vi "Pre Launch Init.vi"(11 "Measurement Señal Actualizable in":refnum<class "Measurement Señal Actualizable.lvclass">) -> (0 "error out":errorcluster, 3 "Measurement Señal Actualizable out":refnum<class "Measurement Señal Actualizable.lvclass">)   [LabVIEW 2020, in "Measurement Señal Actualizable.lvlib" / "Measurement Señal Actualizable.lvclass"]
doc: "(<B>Filename</B>: Actor Framework.lvlib:Actor.lvclass:Pre Launch Init.vi)\n\nDefines behavior that occurs after the Launch Nested Actor method is invoked but before the actor's Actor Core method begins running.\n\nBy default, this method does nothing. A descendant class may override it to define behavior."
uses:
  <vilib>/ActorFramework/Actor/Actor.lvclass
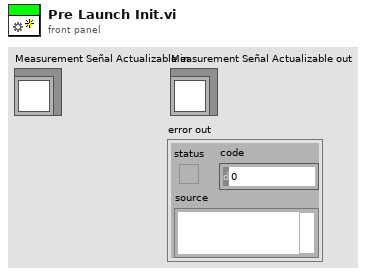
[diagram p1: front panel]
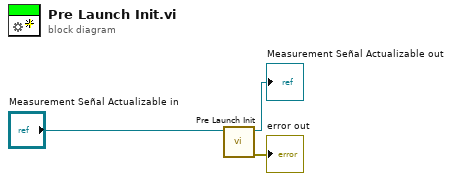
[diagram p0: block diagram]
diagram:
  n1 = call-parent "Pre Launch Init.vi"("Actor in"="Measurement Señal Actualizable in") -> ("error out"=→"error out":errorcluster, "Actor out"=→"Measurement Señal Actualizable out":refnum<class "Measurement Señal Actualizable.lvclass">)  [unwired: 9 in]
